vi "The Need for JTFA.vi"() -> ()   [LabVIEW 2023]
doc: "This example shows the circumstances under which you need time-frequency analysis. For a nonstationary signal, the Fourier transform-based power spectrum may provide useless information or even misleading information. This example illustrates two linear chirp signals. Each signal is a time-reversed version of the other. The power spectrum of the two signals show no differences, while the time-varying frequency contents of the two signals are indicated clearly in the spectrograms.\n\n<b>Instructions:</b>\n1) Run this VI.\n2) Compare the power spectrum and spectrogram of the two signals. Notice how the power spectra are identical, while the spectrograms are different due to the time-varying frequency components."
uses:
  <vilib>/addons/Time Frequency Analysis/typedefs.llb/TFA Data.ctl
  <vilib>/Analysis/4window.llb/windowTd.ctl
  Instance           5 25Saved   The Need for JTFA .vi
  Instance           6 25Saved   The Need for JTFA .vi
  <vilib>/measure/maspectr.llb/FFT Power Spectrum and PSD for 1 Chan.vi
  <vilib>/addons/Time Frequency Analysis/_control.llb/TFA Configure Spectrogram Indicator (Predefined Color Table).vi
  <vilib>/addons/_Advanced Signal Processing/NI_AdvSigProcTFA.lvlib
  <vilib>/Analysis/NI_AALPro.lvlib
  <vilib>/measure/NI_MAPro.lvlib
panel:
  out "aspt-left-top":bool
  out "Power Spectrum of the Reversed Linear Chirp":cluster{"f0":dbl, "df":dbl, "magnitude":dbl[]}(graph)
  out "Power Spectrum of the Linear Chirp":cluster{"f0":dbl, "df":dbl, "magnitude":dbl[]}(graph)
  out "Spectrogram of the Reversed Linear Chirp":dbl[][](graph)
  out "Reversed Linear Chirp":waveform(dbl)(graph)
  out "Spectrogram of the Linear Chirp":dbl[][](graph)
  out "Linear Chirp":waveform(dbl)(graph)
  # "Overview: Shows the circumstances under which you need time-frequency analysis. \nRequirements: LabVIEW Full Development System, Advanced Signal Processing Toolkit\nInstructions: \n1. Run this VI.\n2. Compare the power spectrum and spectrogram of the two signals. Notice how the power spectra are identical, while the spectrograms are different due to the time-varying frequency components."
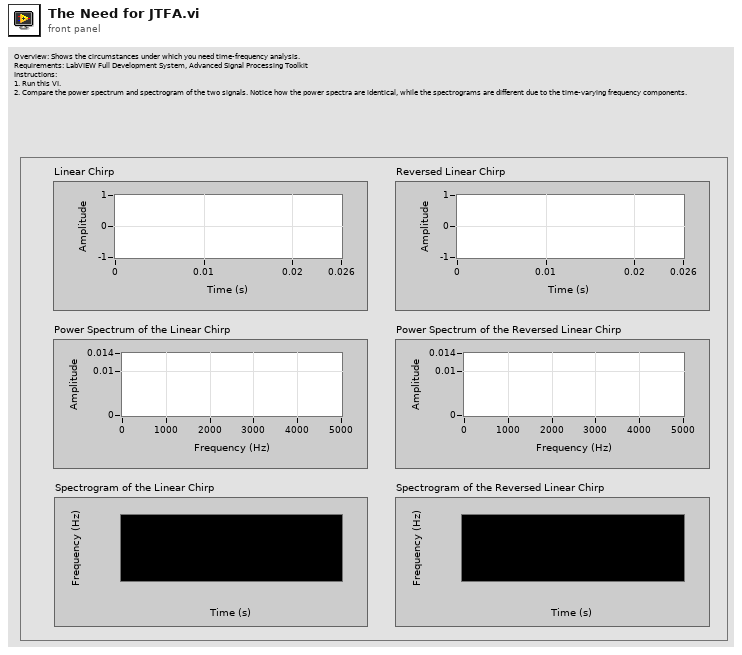
[diagram p1: front panel]
types:
  T1 = typedef "NI_AALPro.lvlib/windowTd.ctl" = u32
  T2 = typedef "NI_AdvSigProcTFA.lvlib/TFA Data.ctl" = u16
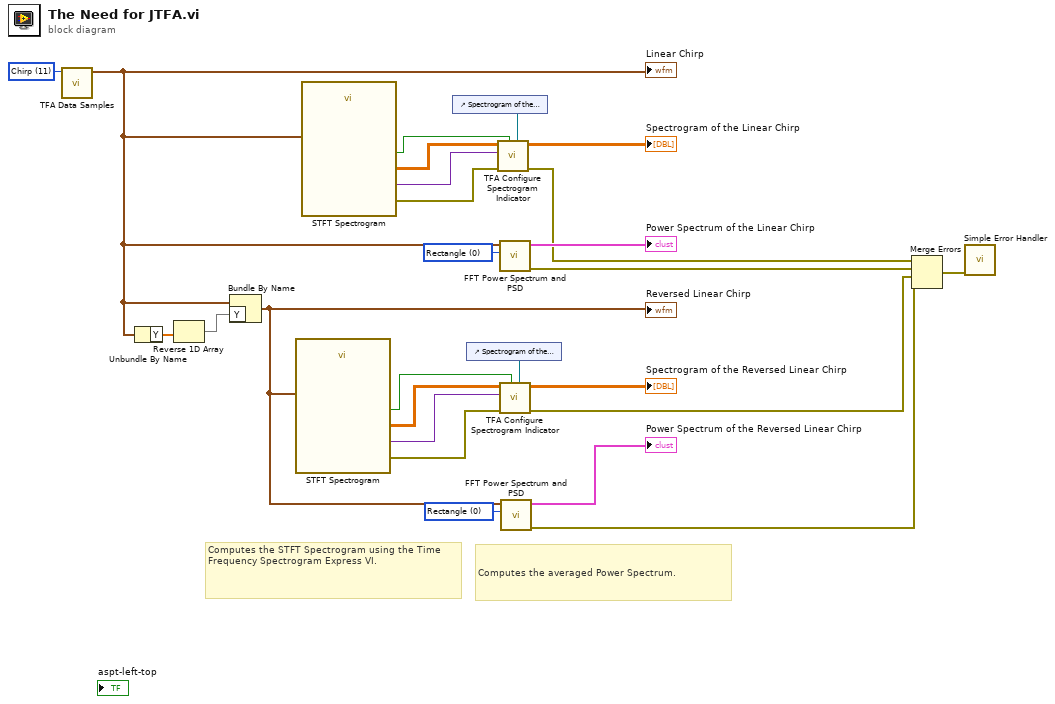
[diagram p0: block diagram]
diagram:
  w8 = T1 0 items=["Rectangle"=0, "Hanning"=1, "Hamming"=2, "Blackman-Harris"=3, "Exact Blackman"=4, "Blackman"=5, "Flat Top"=6, "4 Term B-Harris "=7, "7 Term B-Harris"=8, "Low Sidelobe"=9, "Blackman Nuttall"=11, "Triangle"=30, "Bartlett-Hanning"=31, "Bohman"=32, "Parzen"=33, "Welch"=34, "Kaiser"=60, "Dolph-Chebyshev"=61, "Gaussian"=62] ("window")
  w9 = T1 0 items=["Rectangle"=0, "Hanning"=1, "Hamming"=2, "Blackman-Harris"=3, "Exact Blackman"=4, "Blackman"=5, "Flat Top"=6, "4 Term B-Harris "=7, "7 Term B-Harris"=8, "Low Sidelobe"=9, "Blackman Nuttall"=11, "Triangle"=30, "Bartlett-Hanning"=31, "Bohman"=32, "Parzen"=33, "Welch"=34, "Kaiser"=60, "Dolph-Chebyshev"=61, "Gaussian"=62] ("window")
  w10 = T2 11 items=["PC Fan"=0, "Noisy Chirps"=1, "TDR 1"=2, "TDR 2"=3, "Liquefaction"=4, "Liquefaction Free"=5, "Aneurysm"=6, "Bat"=7, "RF"=8, "Two Gaussian"=9, "Three Gaussian"=10, "Chirp"=11, "Gaussian Chirp"=12, "Cross Chirp"=13, "Doppler"=14, "HOP"=15, "TF Sine"=16, "Three Tone"=17, "Four Tone"=23, "Blood Flow Doppler (phase a)"=20, "Blood Flow Doppler (phase b)"=21, "Heart sound"=22, "-"=18, "Random Noise"=19] ("data")
  # "Computes the averaged Power Spectrum."
  # "Computes the STFT Spectrogram using the Time Frequency Spectrogram Express VI."
  n1 = call <vilib>:"TFA Data Samples.vi"("data"=w10) -> ("signal"=w18:waveform(dbl))  [unwired: 10 out]
  "Linear Chirp" <- w18
  n2 = Unbundle By Name(w18) -> ("Y"=w26:dbl[])
  n3 = Reverse 1D Array(array=w26) -> (reversed array=w25:dbl[])
  n4 = Bundle By Name(cluster=w18, "Y"=w25) -> (w14:waveform(dbl))
  "Reversed Linear Chirp" <- w14
  n5 = call "STFT Spectrogram"("Signal"=w14) -> ("error out"=w6:errorcluster, "Scale Info"=w12:variant, "Spectrogram"=w13:dbl[][], "dB"=w11:bool)  [unwired: 2 in, 5 out]
  n6 = call "STFT Spectrogram"("Signal"=w18) -> ("error out"=w7:errorcluster, "Scale Info"=w16:variant, "Spectrogram"=w17:dbl[][], "dB"=w15:bool)  [unwired: 2 in, 5 out]
  n7 = control-ref of="Spectrogram of the Linear Chirp"() -> (w22:refnum<vi>)
  n8 = control-ref of="Spectrogram of the Reversed Linear Chirp"() -> (w20:refnum<vi>)
  n9 = call-poly <vilib>:"TFA Configure Spectrogram Indicator.vi"("reference of TF spectrogram indicator"=w22, "dB on? (F)"=w15, "error in (no error)"=w7, "scale info"=w16, "spectrogram"=w17) -> ("error out"=w5:errorcluster, "TF spectrogram indicator"=→"Spectrogram of the Linear Chirp":dbl[][])  [unwired: 2 in, 3 out]
  n10 = call-poly <vilib>:"FFT Power Spectrum and PSD.vi"("window"=w8, "time signal"=w18) -> ("error out"=w4:errorcluster, "Power Spectrum / PSD"=→"Power Spectrum of the Linear Chirp":cluster{"f0":dbl, "df":dbl, "magnitude":dbl[]})  [unwired: 6 in, 2 out]
  n11 = call-poly <vilib>:"TFA Configure Spectrogram Indicator.vi"("reference of TF spectrogram indicator"=w20, "dB on? (F)"=w11, "error in (no error)"=w6, "scale info"=w12, "spectrogram"=w13) -> ("error out"=w3:errorcluster, "TF spectrogram indicator"=→"Spectrogram of the Reversed Linear Chirp":dbl[][])  [unwired: 2 in, 3 out]
  n12 = call-poly <vilib>:"FFT Power Spectrum and PSD.vi"("window"=w9, "time signal"=w14) -> ("error out"=w2:errorcluster, "Power Spectrum / PSD"=→"Power Spectrum of the Reversed Linear Chirp":cluster{"f0":dbl, "df":dbl, "magnitude":dbl[]})  [unwired: 6 in, 2 out]
  n13 = Merge Errors(w5, w4, w3, w2) -> (w1:errorcluster)
  n14 = call <vilib>:"Simple Error Handler.vi"("error in (no error)"=w1) -> ()  [unwired: 4 in, 5 out]
